vi "Transfer Controller.vi"(8 "error in":errorcluster) -> ()   [LabVIEW 2025]
doc: "This VI executes continuously carrying out the current operation and responding to updates or new operations. It will often contain the timing or control code that is difficult to place directly in TeleOp. This VI generally opens all sensors and motors and isolates the rest of the robot code from knowing how the operations are carried out."
uses:
  <vilib>/Rock Robotics/WPI/Framework/Completion Status.ctl
  Transfer Setpoints.ctl
  Transfer Operations.ctl
  <vilib>/Rock Robotics/WPI/ThirdParty/REV Robotics/REVLib/Typedef/SPARK Feed Forward Gains.ctl
  <vilib>/Rock Robotics/WPI/ThirdParty/REV Robotics/REVLib/Typedef/Spark MAX Idle Mode.ctl
  <vilib>/Rock Robotics/WPI/ThirdParty/REV Robotics/REVLib/Typedef/Spark MAX Control Type.ctl
  cd766d12-11c7-4c29-bbba-655644d1f119.vi
  6021059d-2c14-4f91-8428-3fe9424e4eb1.vi
  <vilib>/Rock Robotics/WPI/ThirdParty/REV Robotics/REVLib/SubVI/Public/SPARK Open Brushless.vi
  <vilib>/Rock Robotics/WPI/ThirdParty/REV Robotics/REVLib/SubVI/Public/SPARK Configure Basic Idle Mode.vi
  <vilib>/Rock Robotics/WPI/ThirdParty/REV Robotics/REVLib/SubVI/Public/SPARK Get Encoder Status Velocity.vi
  Framework/Robot Global Data.vi
  <vilib>/Rock Robotics/Network Tables/NT Write Boolean.vi
panel:
  in  "Transfer Gains":T2={{"P Gain"=3.0000000000000004e-05, "I Gain"=0.0, "D Gain"=0.0}, "Feed Forward Gains"={"kV"=0.0019, "kS"=0.0, "kA"=0.0, "kG"=0.0, "kCos"=0.0, "kCosRatio"=0.0}, "I Zone"=0.0, "Min Output"=-0.95, "Max Output"=0.95}
  out "Transfer Velocity":T3(graph)
  out "LPK Velocity":T3(graph)={"Transfer Speed"=5000.0, "Sensor Velocity"=4962.12890625}
  in  "Kicker Gains":T2={{"P Gain"=0.00040000000000000013, "I Gain"=0.0, "D Gain"=0.007}, "Feed Forward Gains"={"kV"=0.00175, "kS"=0.0, "kA"=0.0, "kG"=0.0, "kCos"=0.0, "kCosRatio"=0.0}, "I Zone"=0.0, "Min Output"=-0.95, "Max Output"=0.95}
  in  "Interactive Values":T4
  out "Current\nCmd":string="Started at  00:33:37.761\nReserve: Reserve,  S 0.0, D 0.000000"
  in  "Buttons":cluster{"Execute Cmd":bool, "Abort Cmd":bool}
  out "Command Timing":cluster{"Start Time (ms)":u32, "Iterations":i32}={"Start Time (ms)"=660026, "Iterations"=0}
  out "Status":T6=enum."Aborted"
  # "Tip: It may be helpful to observe inputs and sensor values.\nYou may also want to display tuning or debugging controls."
  # "Interactive Command: You may fill in the settings for a command\nand schedule it with the Execute button. You can observe and abort\nany command while fine tuning the code for the controller."
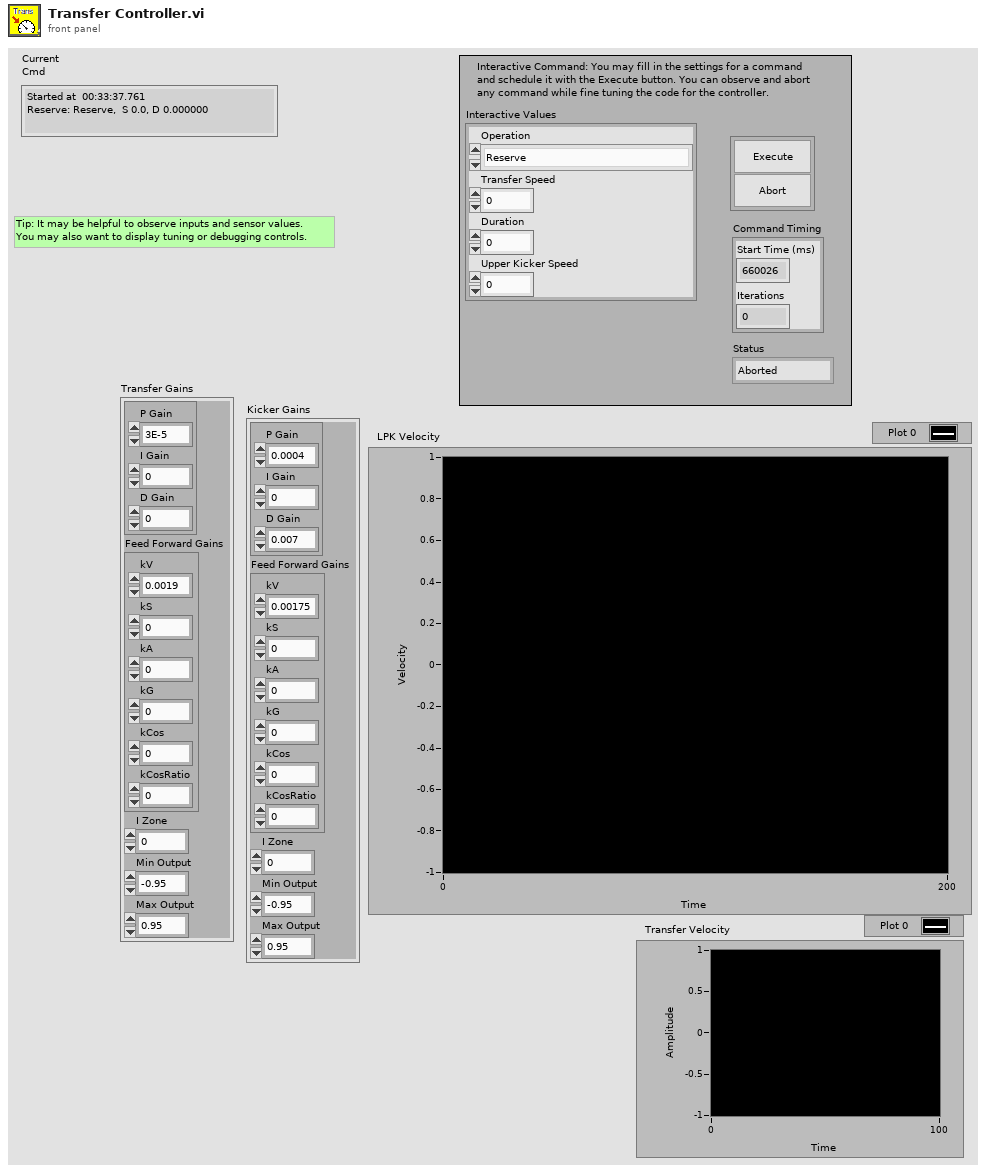
[diagram p1: front panel]
types:
  T1 = typedef "SPARK Feed Forward Gains.ctl" = cluster{"kV":dbl, "kS":dbl, "kA":dbl, "kG":dbl, "kCos":dbl, "kCosRatio":dbl}
  T2 = cluster{cluster{"P Gain":dbl, "I Gain":dbl, "D Gain":dbl}, "Feed Forward Gains":T1, "I Zone":dbl, "Min Output":dbl, "Max Output":dbl}
  T3 = cluster{"Transfer Speed":dbl, "Sensor Velocity":dbl}
  T4 = typedef "Transfer Setpoints.ctl" = cluster{"Operation":T5, "Transfer Speed":dbl, "Duration":dbl, "Upper Kicker Speed":dbl}
  T5 = typedef "Transfer Operations.ctl" = enum16{"Reserve", "Read Current", "Immediate"}
  T6 = typedef "Completion Status.ctl" = enum16{"Successful", "Aborted", "Incomplete"}
  T7 = typedef "Spark MAX Idle Mode.ctl" = enum16{"Coast", "Brake"}
  T8 = typedef "WPI_MotorControlDeviceRef.ctl" = cluster{"DeviceStatus":errorcluster, "Type":T9, "PWM":cluster{"PWM Channel":T10, "DeadBand":T11}, "CAN":cluster{"Device Number":u8, "SetOutput VI Ref":variant, "GetOutput VI Ref":variant, "Enable VI Ref":variant, "Disable VI Ref":variant, "Data":variant}, "Invert":bool, "DIO PWM":cluster{"PWM \"Enable\" Channel":T10, "DIOChannel":T12, "PWM Rate":dbl}}
  T9 = typedef "WPI_MotorControlType.ctl" = enum16{"PWM", "CAN", "DIO PWM"}
  T10 = typedef "FPGA_DIOPWMChannel.ctl" = enum8{"PWM 0", "PWM 1", "PWM 2", "PWM 3", "PWM 4", "PWM 5", "PWM 6", "PWM 7", "PWM 8", "PWM 9", "PWM MXP 0", "PWM MXP 1", "PWM MXP 2", "PWM MXP 3", "PWM MXP 4", "PWM MXP 5", "PWM MXP 6", "PWM MXP 7", "PWM MXP 8", "PWM MXP 9", "Invalid"}
  T11 = typedef "WPI_PWMDeadband.ctl" = cluster{"Name":string, "maxPositivePwm":i32, "minPositivePwm":i32, "centerPwm":i32, "maxNegativePwm":i32, "minNegativePwm":i32, "angularRange":u16}
  T12 = typedef "FPGA_DIOChannel.ctl" = enum8{"DIO 0", "DIO 1", "DIO 2", "DIO 3", "DIO 4", "DIO 5", "DIO 6", "DIO 7", "DIO 8", "DIO 9", "DIO MXP 0", "DIO MXP 1", "DIO MXP 2", "DIO MXP 3", "DIO MXP 4", "DIO MXP 5", "DIO MXP 6", "DIO MXP 7", "DIO MXP 8", "DIO MXP 9", "DIO MXP 10", "DIO MXP 11", "DIO MXP 12", "DIO MXP 13", "DIO MXP 14", "DIO MXP 15", "SPI Port CS1", "SPI Port CS2", "SPI Port CS3", "SPI Port MISO", "SPI Port MOSI", "Invalid"}
  T13 = typedef "Command Status Info.ctl" = cluster{"Name":string, "Status":T6, "notifier out":T14}
  T14 = typedef "Completion Notifier.ctl" = refnum<notifier>
  T15 = cluster{"Current Command":T4, "Command Timing":cluster{"Start Time (ms)":u32, "Iterations":i32}, "Command Arguments":cluster{"Command Info":T13, "Description":string, "Default Command":T4, "queue out":refnum<queue>, "Subsystem Name":string}}
  T16 = typedef "Spark MAX Control Type.ctl" = enum16{"Percent VBus", "Voltage", "Velocity", "Position", "Smart Motion", "Current", "Smart Velocity", "MAXMotion Position", "MAXMotion Velocity"}
  T17 = typedef "WPI_DriverStationRobotMode2.ctl" = enum16{"Autonomous Disabled", "Autonomous Enabled", "Teleop Disabled", "Teleop Enabled", "Disconnected", "Finish", "Test Disabled", "Test Enabled", "Emergency Stopped"}
  T18 = cluster{"Upper Kicker Speed":dbl, "Sensor Velocity":dbl}
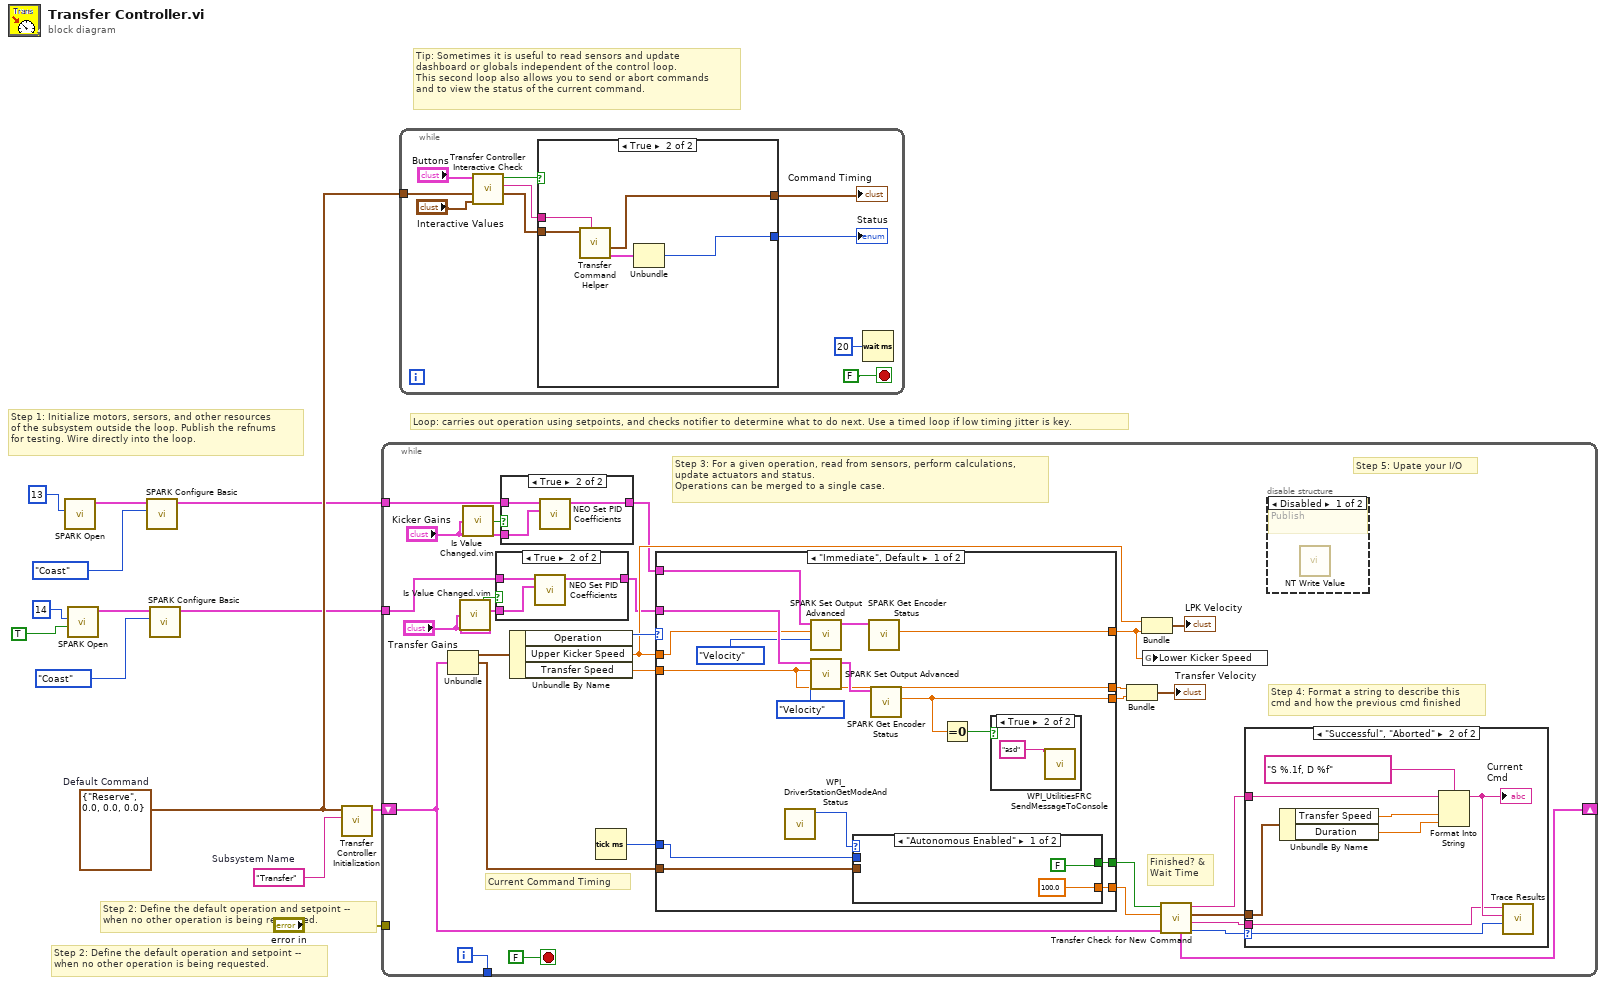
[diagram p0: block diagram]
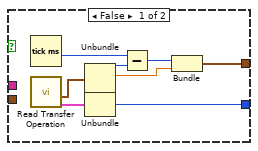
[diagram p2: hidden frame]
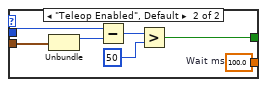
[diagram p8: hidden frame]
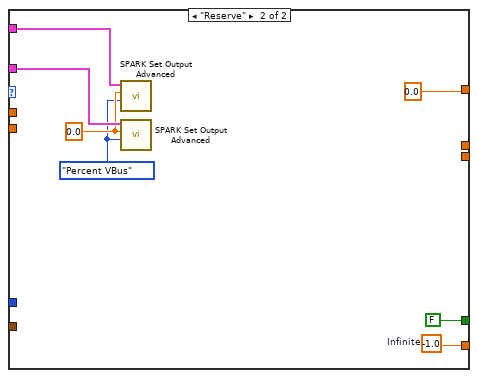
[diagram p9: hidden frame]
diagram:
  w10 = T4 {"Operation"=enum."Reserve", "Transfer Speed"=0.0, "Duration"=0.0, "Upper Kicker Speed"=0.0}  # Default Command
  w11 = "Transfer"  # Subsystem Name
  # "Step 2: Define the default operation and setpoint --\nwhen no other operation is being requested."
  # "Tip: Sometimes it is useful to read sensors and update\ndashboard or globals independent of the control loop.\nThis second loop also allows you to send or abort commands\nand to view the status of the current command."
  # "Step 2: Define the default operation and setpoint --\nwhen no other operation is being requested."
  # "Step 1: Initialize motors, sersors, and other resources\nof the subsystem outside the loop. Publish the refnums\nfor testing. Wire directly into the loop."
  # "Loop: carries out operation using setpoints, and checks notifier to determine what to do next. Use a timed loop if low timing jitter is key."
  n1 = call-poly <vilib>:"SPARK Open.vi"("Device Number"=u8 13) -> ("MotorControlDeviceRef"=w9:T8)  [unwired: 9 in, 1 out]
  n2 = call-poly <vilib>:"SPARK Open.vi"("Invert"=TRUE, "Device Number"=u8 14) -> ("MotorControlDeviceRef"=w4:T8)  [unwired: 8 in, 1 out]
  n3 = call-poly <vilib>:"SPARK Configure Basic.vi"("Idle Mode"=Spark_MAX_Idle_Mode."Coast", "MotorControlDeviceRef in"=w9) -> ("MotorControlDeviceRef out"=w6:T8)  [unwired: 8 in, 1 out]
  n4 = call-poly <vilib>:"SPARK Configure Basic.vi"("Idle Mode"=Spark_MAX_Idle_Mode."Coast", "MotorControlDeviceRef in"=w4) -> ("MotorControlDeviceRef out"=w5:T8)  [unwired: 8 in, 1 out]
  n5 = call "Transfer Controller Initialization.vi"("Subsystem Name"=w11, "Default Command"=w10) -> ("Current Command"=w12:T15)  [unwired: 9 in]
  n6 = while {
    shift-right: [w34] -> _
    shift-left: w12 -> [w27]
    tunnel: [w41] -> _
    tunnel: "error in" -> [_]
    tunnel: w6 -> [w23]
    tunnel: w5 -> [w17]
    i -> [w41]
    stop <- FALSE stop-if-true
    # "Step 5: Upate your I/O"
    # "Step 4: Format a string to describe this\ncmd and how the previous cmd finished"
    # "Current Command Timing"
    # "Finished? &\nWait Time"
    # "Step 3: For a given operation, read from sensors, perform calculations,\nupdate actuators and status.\nOperations can be merged to a single case."
    n7 = Unbundle(w27) -> ("Current Command"=w40:T4, "Command Timing"=w36:cluster{"Start Time (ms)":u32, "Iterations":i32})  [unwired: 1 out]
    n8 = call "Is Value Changed.vim"("value"="Transfer Gains") -> ("changed or first call?"=w15:bool)
    n9 = call "Is Value Changed.vim"("value"="Kicker Gains") -> ("changed or first call?"=w25:bool)
    n10 = case shown="True" w15 {
      tunnel: w17 -> [w43 w46]
      tunnel: [w43 w45] -> w16
      tunnel: "Transfer Gains" -> [_ w44]
      frame False {
      }
      frame True {
        n11 = call "NEO Set PID Coefficients.vi"("PID Gains"=w44, "MotorControlDeviceRef in"=w46) -> ("MotorControlDeviceRef out"=w45:T8)  [unwired: 6 in, 1 out]
      }
    }
    n12 = case shown="True" w25 {
      tunnel: w23 -> [w47 w50]
      tunnel: [w47 w49] -> w24
      tunnel: "Kicker Gains" -> [_ w48]
      frame False {
      }
      frame True {
        n13 = call "NEO Set PID Coefficients.vi"("PID Gains"=w48, "MotorControlDeviceRef in"=w50) -> ("MotorControlDeviceRef out"=w49:T8)  [unwired: 6 in, 1 out]
      }
    }
    n14 = Unbundle By Name(w40) -> ("Operation"=w39:T5, "Upper Kicker Speed"=w38:dbl, "Transfer Speed"=w35:dbl)
    n15 = Tick Count (ms)() -> (millisecond timer value=w37:u32)
    n16 = case shown="\"Immediate\", Default" w39 {
      tunnel: [w66 w91] -> w32
      tunnel: [w67 FALSE ("ignore previous (F)")] -> w33
      tunnel: w36 -> [w64 _]
      tunnel: w38 -> [w70 _]
      tunnel: w37 -> [w65 _]
      tunnel: w35 -> [w61 _]
      tunnel: w24 -> [w74 w88]
      tunnel: w16 -> [w73 w89]
      tunnel: [w63 0.0 ("Sensor Velocity")] -> w21
      tunnel: [w60 _] -> w20
      tunnel: [w61 _] -> w18
      frame "Immediate", Default {
        n17 = call <vilib>:"WPI_DriverStationGetModeAndStatus.vi"() -> ("Robot Mode"=w68:T17)  [unwired: 10 in, 1 out]
        n18 = call <vilib>:"SPARK Set Output Advanced.vi"("Control Mode"=Spark_MAX_Control_Type."Velocity", "Setpoint"=w70, "MotorControlDevRef"=w74) -> ("MotorControlDevRef"=w69:T8)  [unwired: 7 in, 1 out]
        n19 = call <vilib>:"SPARK Set Output Advanced.vi"("Control Mode"=Spark_MAX_Control_Type."Velocity", "Setpoint"=w61, "MotorControlDevRef"=w73) -> ("MotorControlDevRef"=w62:T8)  [unwired: 7 in, 1 out]
        n20 = case shown="\"Autonomous Enabled\"" w68 {
          tunnel: [100.0 ("Wait ms") w84] -> w66
          tunnel: w64 -> [_ w80]
          tunnel: w65 -> [_ w79]
          tunnel: [FALSE w78] -> w67
          frame "Autonomous Enabled" {
          }
          frame "Teleop Enabled", Default {
            w84 = 100.0  # Wait ms
            n21 = Unbundle(w80) -> ("Start Time (ms)"=w83:u32)  [unwired: 1 out]
            n22 = Subtract(x=w79, y=w83) -> (x-y=w82:u32)
            n23 = Greater?(x=w82, y=u8 50 ("Left Motor")) -> (0:w78:bool)
          }
        }
        n24 = call-poly <vilib>:"SPARK Get Encoder Status.vi"("MotorControlDevRef in"=w69) -> ("Sensor Velocity"=w63:dbl)  [unwired: 7 in, 3 out]
        n25 = call-poly <vilib>:"SPARK Get Encoder Status.vi"("MotorControlDevRef in"=w62) -> ("Sensor Velocity"=w60:dbl)  [unwired: 7 in, 3 out]
        n26 = Equal To 0?(x=w60) -> (x = 0?=w59:bool)
        n27 = case shown="True" w59 {
          frame False {
          }
          frame True {
            n28 = call <vilib>:"WPI_UtilitiesFRC SendMessageToConsole.vi"("Message"="asd") -> ()  [unwired: 14 in, 1 out]
          }
        }
      }
      frame "Reserve" {
        w87 = 0.0 ("Setpoint")
        w86 = Spark_MAX_Control_Type."Percent VBus" ("Control Mode")
        w91 = -1.0  # Infinite
        n29 = call <vilib>:"SPARK Set Output Advanced.vi"("Control Mode"=w86, "Setpoint"=w87, "MotorControlDevRef"=w88) -> ()  [unwired: 7 in, 2 out]
        n30 = call <vilib>:"SPARK Set Output Advanced.vi"("Control Mode"=w86, "Setpoint"=w87, "MotorControlDevRef"=w89) -> ()  [unwired: 7 in, 2 out]
      }
    }
    n31 = Bundle("Transfer Speed"=w18, "Sensor Velocity"=w20) -> (→"Transfer Velocity":T3)  [unwired: 1 in]
    n32 = Bundle("Upper Kicker Speed"=w38, "Sensor Velocity"=w21) -> (→"LPK Velocity":T18)  [unwired: 1 in]
    n33 = global write "Robot Global Data.vi" "Lower Kicker Speed"(w21) -> ()
    n34 = call "Transfer Check for New Command.vi"("Current Command"=w27, "Wait time (ms)"=w32, "Finished?"=w33) -> ("Completion"=w28:T6, "Subsystem Name"=w29:string, "Current Command"=w30:T4, "Initial Trace String"=w31:string, "NextCommand"=w34:T15)  [unwired: 4 in]
    n35 = case shown="\"Successful\", \"Aborted\"" w28 {
      selector: w28 -> [_ w58]
      tunnel: w31 -> [_ w54]
      tunnel: w30 -> [_ w55]
      tunnel: w29 -> [_ w51]
      frame "Incomplete", Default {
        # "Continuing current command"
      }
      frame "Successful", "Aborted" {
        # "Report and setup for next command"
        n36 = Unbundle By Name(w55) -> ("Transfer Speed"=w57:dbl, "Duration"=w52:dbl)
        n37 = Format Into String(format string="S %.1f, D %f", initial string=w54, w57, w52) -> (resulting string=w53:string)  [unwired: 1 in, 1 out]
        "Current\nCmd" <- w53
        n38 = call <vilib>:"Trace Results.vi"("Status of previous command"=w58, "Description"=w53, "Subsystem"=w51) -> ()  [unwired: 9 in]
      }
    }
    n39 = disable-structure shown="Disabled" {
      frame Disabled {
        # "Publish"
        n40 = call-poly <vilib>:"NT Write Value.vi"() -> ()  [unwired: 11 in, 1 out]
      }
      frame Enabled {
      }
    }
  }
  n41 = while {
    tunnel: w10 -> [w98]
    stop <- FALSE stop-if-true
    n42 = call "Transfer Controller Interactive Check.vi"("Interactive Command in"="Interactive Values", "Default Command"=w98, "Buttons"="Buttons") -> ("Interactive Command out"=w95:T4, "Trace String"=w96:string, "Schedule"=w97:bool)  [unwired: 6 in]
    n43 = case shown="True" w97 {
      tunnel: [w109 w114] -> w94
      tunnel: w95 -> [_ w112]
      tunnel: [w105 w110] -> w93
      tunnel: w96 -> [_ w113]
      frame False {
        n44 = Tick Count (ms)() -> (millisecond timer value=w104:u32)
        n45 = call "Read Transfer Operation.vi"() -> ("Command Info"=w102:T13, "SubSystem Data"=w103:T4)  [unwired: 9 in, 1 out]
        n46 = Unbundle(w103) -> ("Operation"=w108:T5, "Transfer Speed"=w106:dbl)  [unwired: 2 out]
        n47 = Unbundle(w102) -> ("Status"=w109:T6)  [unwired: 2 out]
        n48 = Subtract(x=w104, y=w108) -> (x-y=w107:u32)
        n49 = Bundle(w107, "Transfer Speed"=w106) -> (w105:cluster{u32, "Transfer Speed":dbl})  [unwired: 1 in]
      }
      frame True {
        n50 = call "Transfer Command Helper.vi"("Description"=w113, "SubSystem Data"=w112) -> ("Command Info Out"=w111:T13, "Command Timing"=w110:cluster{"Start Time (ms)":u32, "Iterations":i32})  [unwired: 7 in, 1 out]
        n51 = Unbundle(w111) -> ("Status"=w114:T6)  [unwired: 2 out]
      }
    }
    "Status" <- w94
    "Command Timing" <- w93
    n52 = Wait (ms)(milliseconds to wait=u32 20) -> ()  [unwired: 1 out]
  }
